vi "Main.vi"() -> ()   [LabVIEW 2021, in "Sound Manager.lvlib"]
uses:
  Sound Manager.lvlib
  Typedefs/Sound Effects.ctl
  Typedefs/States.ctl
  Typedefs/Config.ctl
  <vilib>/sound2/lvsound2.llb/Sound Output Task ID.ctl
  <vilib>/event_ctls.llb/usereventprio.ctl
  Application/App Configuration.ctl
  Application/Application.lvclass
  Configuration/Configuration.lvlib
  SubVIs/Read Sound ConfigurationI.vi
panel:
  in  "Multicolumn Listbox":i32(listbox)
  out "Background Track":string
  in  "Stop Sound Effect":bool
  in  "Play Sound Effect":bool
  in  "Sound Effect":T1
  in  "Background music":bool
  in  "Load Config":bool
  in  "Module_Refs":T2={"ModuleName"=enum."Controller", "Queue"=refnum, "user event"=refnum, "VI Refnum"=refnum, "ShowFP"=FALSE, "StatesTracking Enabled"=FALSE}
  out "error out":errorcluster
  in  "error in (no error)":errorcluster
  out "Message":string
  in  "Stop App":bool
  in  "Stop Module":bool
  # "#Architecture\n\nPlace inside this box all visible data."
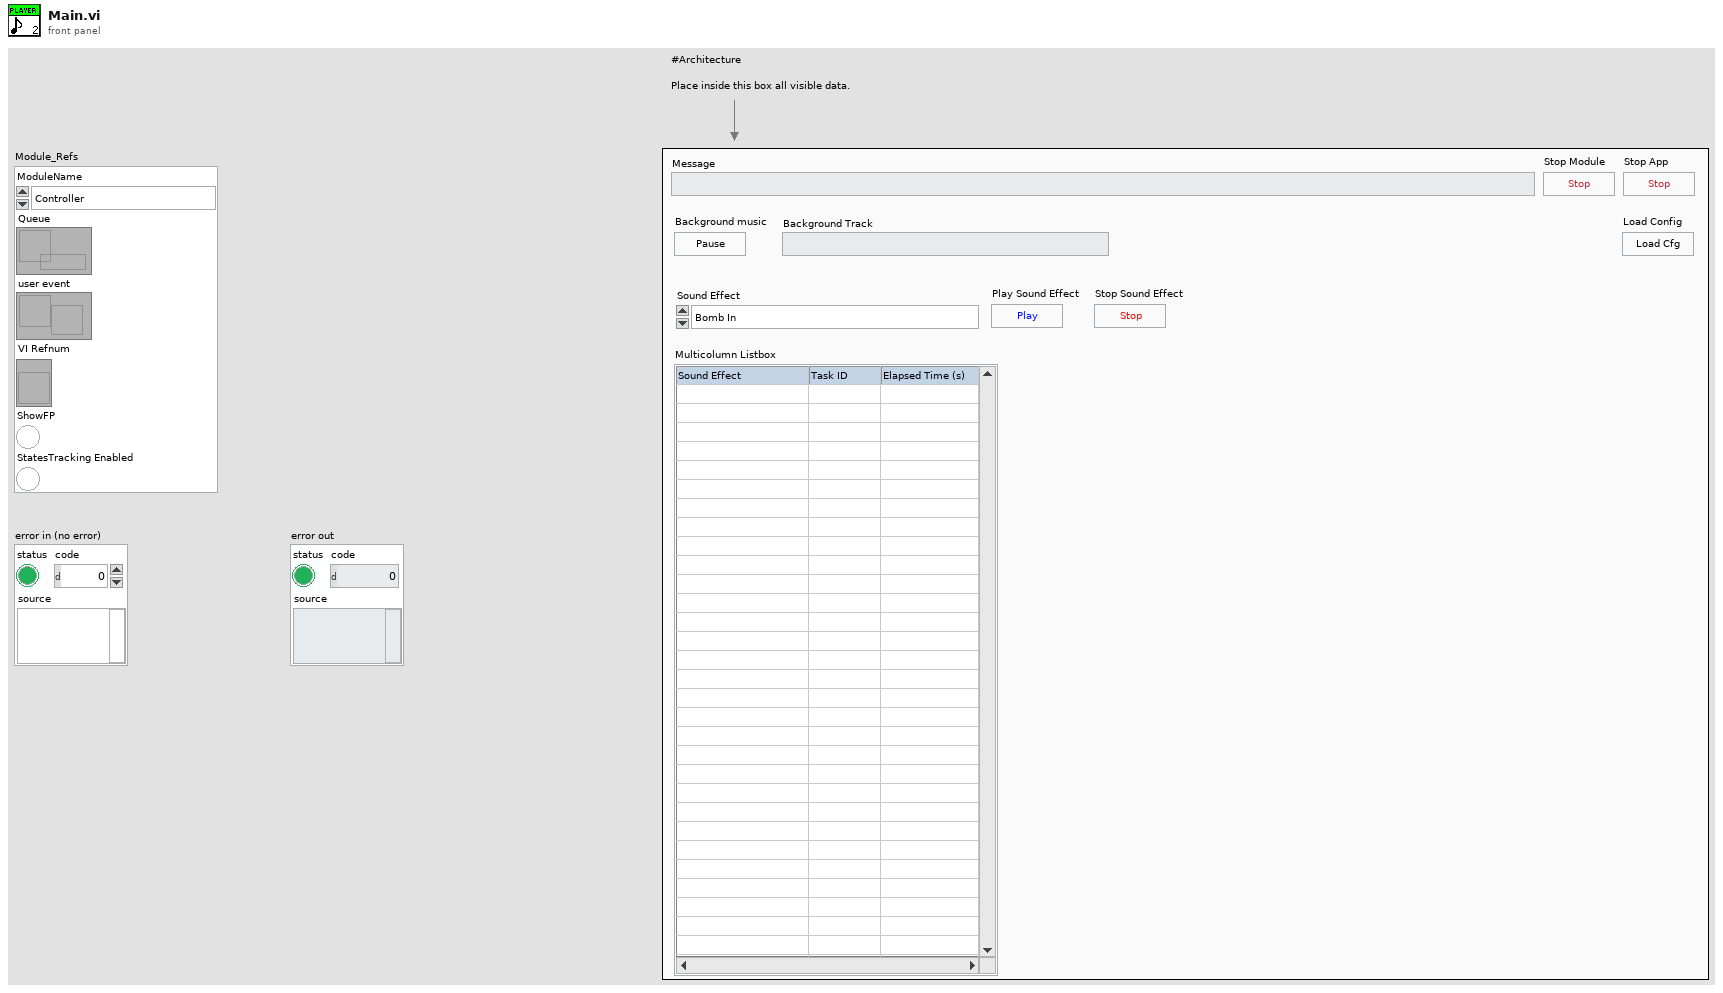
[diagram p1: front panel]
types:
  T1 = typedef "Sound Manager.lvlib/Sound Effects.ctl" = enum16{"Bomb In", "Bomb Out", "Bomb Touched", "Game Over", "Victory", "Eat", "10 Fruits", "Eat2", "Eat3", "Eat4", "MaxShield", "Shield", "10p", "Grape In", "Grape Out", "20p", "30p", "40p", "50p", "60p", "70p", "80p", "90p", "100p", "All shields cracked", "Mouse In", "Mouse Out", "Mouse Eaten", "Grape Eaten", "States Recover", "Broken Shield", "Bonus", "Happy Time", "explode", "Game over musica", "Back Music", "Shield Catch", "Evil lough", "Cricket In", "Cricket eaten", "Lets Go", "Jump1", "Jump2", "Jump3", "Unstoppable", "Troll Music", "winner"}
  T2 = typedef "Architecture.lvlib/Module References.ctl" = cluster{"ModuleName":T3, "Queue":refnum<queue>, "user event":refnum<user-event>, "VI Refnum":refnum<vi>, "ShowFP":bool, "StatesTracking Enabled":bool}
  T3 = typedef "Architecture.lvlib/Enum_Module_Name.ctl" = enum16{"Configuration", "Error_Handler", "Log", "Database", "Controller"}
  T4 = typedef "Sound Manager.lvlib/States.ctl" = cluster{"Module_Refs":T2, "Response Data":variant, "Config":T5, "Music Paused":bool, "Tasks":cluster{"Sound Effect":T1, "Task ID":T6, "Init":timestamp}[]}
  T5 = typedef "Sound Manager.lvlib/Config.ctl" = cluster{"Sound Library Path":path, "dyn sounds path":path}
  T6 = typedef "Sound Output Task ID.ctl" = u32
  T7 = enum32{"Invalid", "Standard", "Closed", "Hidden", "Minimized", "Maximized"}
  T8 = typedef "Error_Manager.lvlib/LogRotate.lvclass/LogData.ctl" = cluster{"error in":errorcluster, "replacements":string[], "Time Stamp":timestamp}
  T9 = cluster{"Sound Effect":T1, "Task ID":T6, "Init":timestamp}[]
  T10 = cluster{"Sound Effect":T1, "Task ID":T6, "Init":timestamp}
  T11 = typedef "usereventprio.ctl" = enum32{"high priority", "normal priority"}
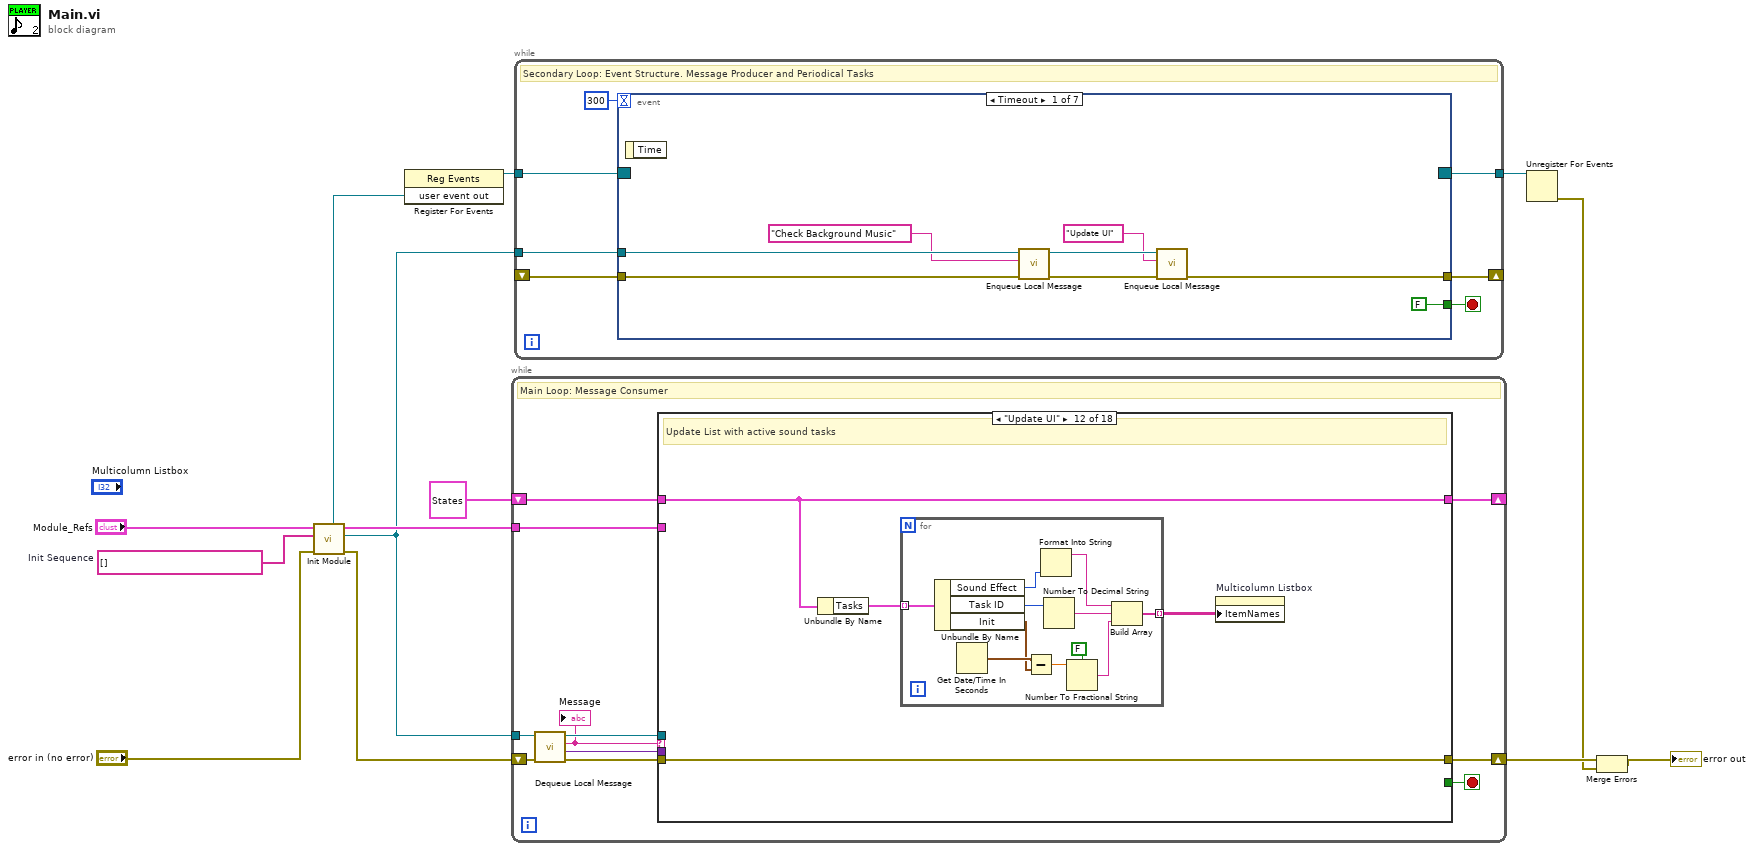
[diagram p0: block diagram]
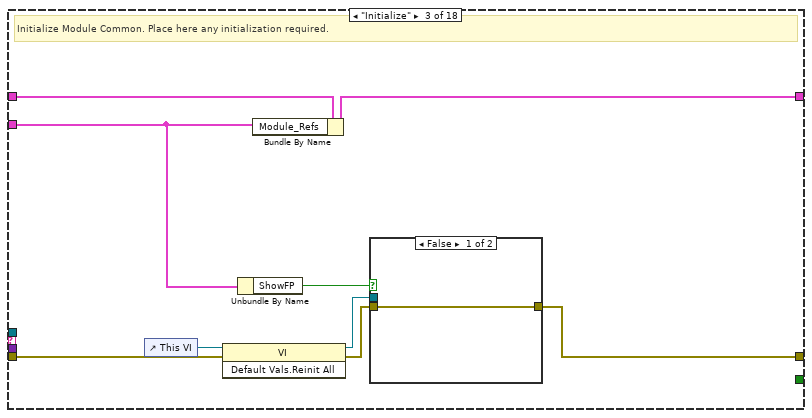
[diagram p4: hidden frame]
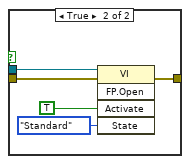
[diagram p5: hidden frame]
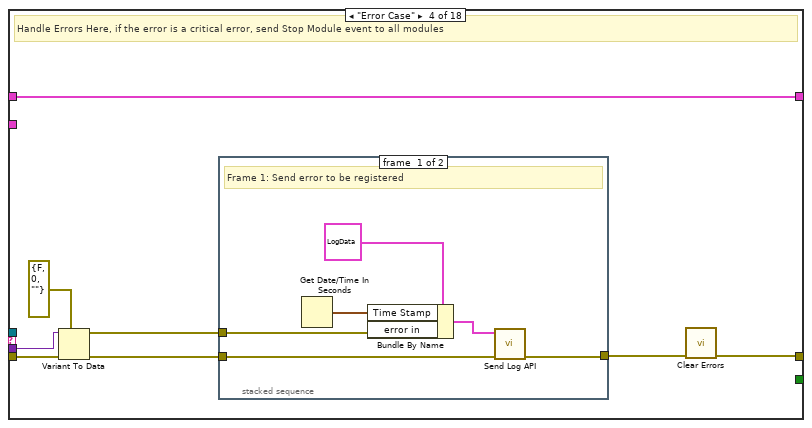
[diagram p6: hidden frame]
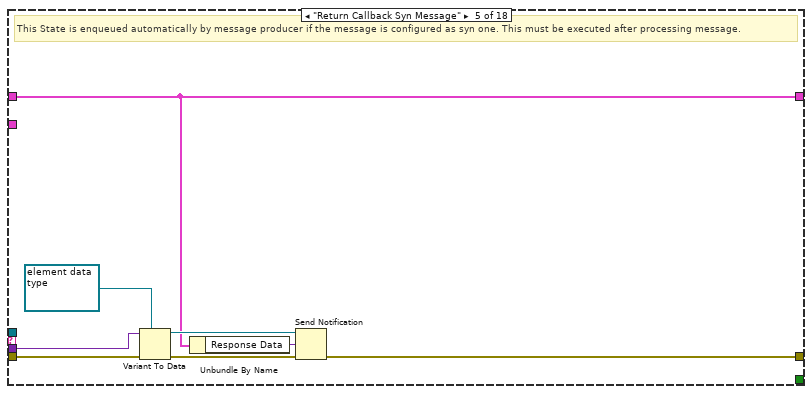
[diagram p9: hidden frame]
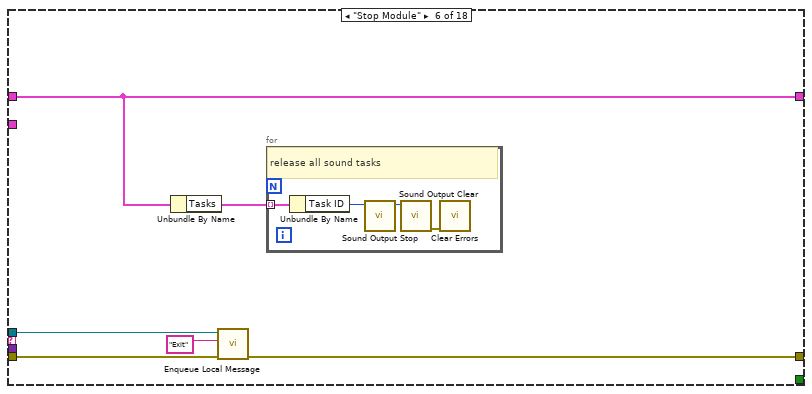
[diagram p10: hidden frame]
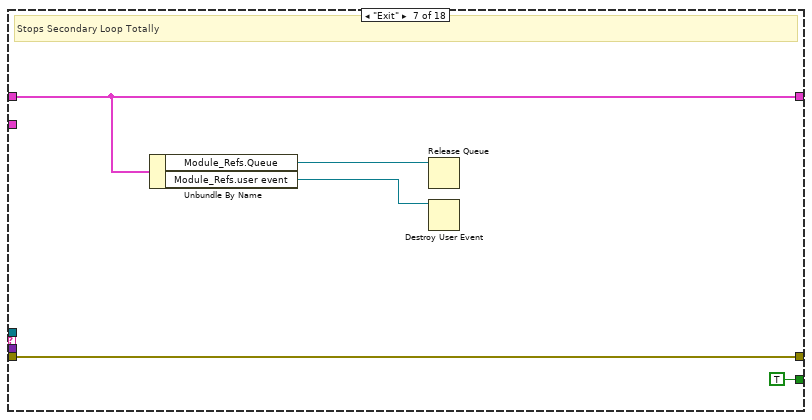
[diagram p11: hidden frame]
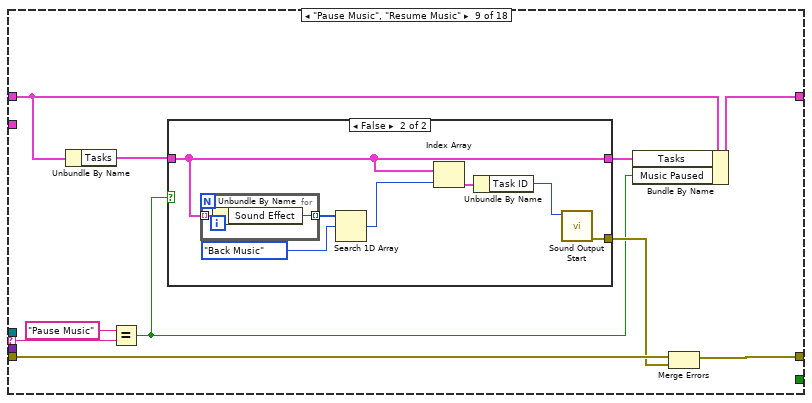
[diagram p13: hidden frame]
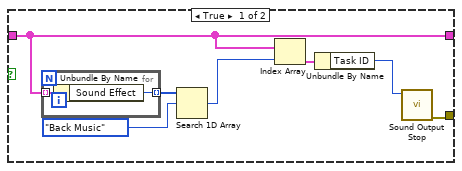
[diagram p14: hidden frame]
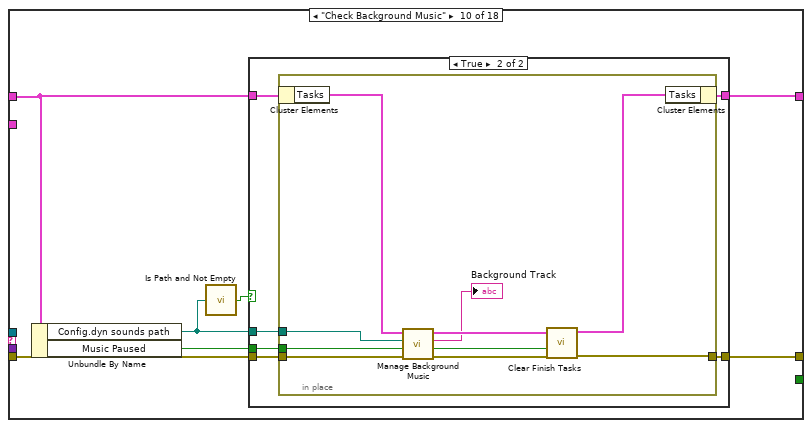
[diagram p15: hidden frame]
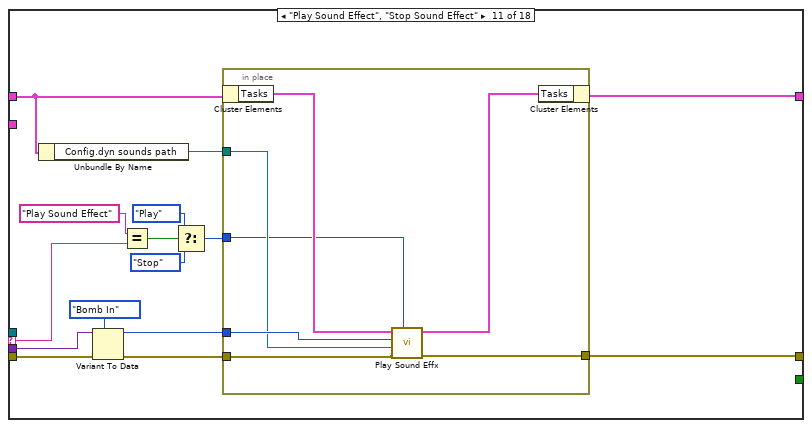
[diagram p17: hidden frame]
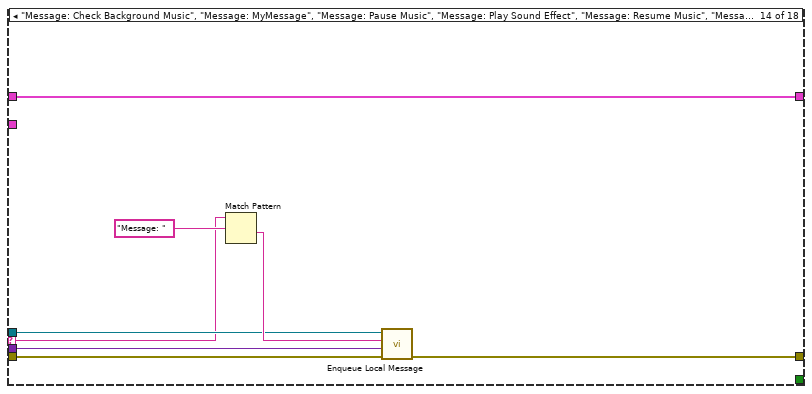
[diagram p19: hidden frame]
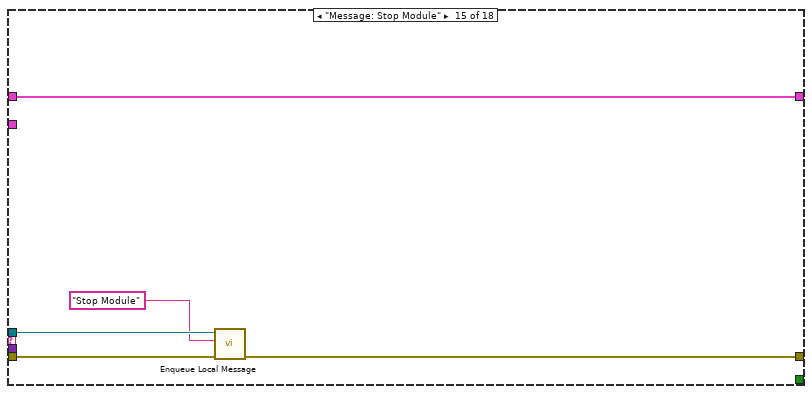
[diagram p20: hidden frame]
diagram:
  w11 = string[] []  # Init Sequence
  n1 = call "Init Module.vi"("error in (no error)"="error in (no error)", "Init Sequence"=w11, "Module Refs"="Module_Refs") -> ("error out"=w13:errorcluster, "queue out"=w2:refnum<queue>, "Module Refs Out"=w4:T2, "user event out"=w3:refnum<user-event>)  [unwired: 5 in]
  n2 = register-events(w3) -> (reference out=w10:refnum<event-registration>)  [unwired: 2 in, 1 out]
  n3 = while {
    shift-right: [w23] -> _
    shift-left: T4 {"Module_Refs"={"ModuleName"=enum."Controller", "Queue"=refnum, "user event"=refnum, "VI Refnum"=refnum, "ShowFP"=FALSE, "StatesTracking Enabled"=FALSE}, "Response Data"=variant, "Config"={"Sound Library Path"=path "", "dyn sounds path"=path ""}, "Music Paused"=FALSE, "Tasks"=[]} ("SM Data") -> [w24]
    shift-right: [w22] -> w8
    shift-left: w13 -> [w20]
    tunnel: w2 -> [w21]
    tunnel: w4 -> [w14]
    stop <- w15 stop-if-true
    # "Main Loop: Message Consumer"
    n4 = call "Dequeue Local Message.vi"("error in"=w20, "Msg queue in"=w21) -> ("error out"=w19:errorcluster, "Data"=w16:variant, "Message"=w17:string, "queue out"=w18:refnum<queue>)  [unwired: 6 in]
    "Message" <- w17
    n5 = case shown="\"Update UI\"" w17 {
      selector: w17 -> [_ _ _ _ _ _ _ _ w94 _ w144 _ _ w178 _ _ _ w222]
      tunnel: w24 -> [w26 w28 w37 w51 w63 w71 w82 w86 w92 w118 w148 w163 w177 w185 w190 w195 w213 w227]
      tunnel: [w26 w28 w35 w51 w63 w71 w82 w86 w95 w117 w146 w163 w177 w185 w190 w191 w213 w227] -> w23
      tunnel: w19 -> [w25 w27 w36 w50 w69 w75 w84 w85 w96 w120 w153 w164 w176 w182 w189 w194 w212 w226]
      tunnel: [w25 w27 w31 w44 w68 w74 w84 w85 w89 w119 w145 w164 w176 w179 w188 w192 w212 w216] -> w22
      tunnel: w18 -> [_ _ _ _ _ w73 _ _ _ _ _ _ _ w180 w187 _ _ w223]
      tunnel: w16 -> [_ _ _ w49 w66 _ _ _ _ _ w152 _ _ w181 _ w193 _ w224]
      tunnel: [_ _ _ _ _ _ TRUE _ _ _ _ _ _ _ _ _ _ _] -> w15
      tunnel: w14 -> [_ _ w34 _ _ _ _ _ _ _ _ _ _ _ _ _ _ _]
      frame "--------State Machine Arquitechture Operations--------" {
      }
      frame "Idle", Default {
        # "Use this state to make iterations if required."
      }
      frame "Initialize" {
        # "Initialize Module Common. Place here any initialization required."
        n6 = control-ref of="This VI"() -> (w29:refnum<vi>)
        n7 = invoke class="VI" method="Default Vals.Reinit All"(reference=w29, error in=w36) -> (reference out=w32:refnum<vi>, error out=w33:errorcluster)  [unwired: 1 in, 1 out]
        n8 = Unbundle By Name(w34) -> ("ShowFP"=w30:bool)
        n9 = Bundle By Name(cluster=w37, "Module_Refs"=w34) -> (w35:T4)
        n10 = case shown="False" w30 {
          tunnel: w33 -> [w38 w43]
          tunnel: [w38 w42] -> w31
          tunnel: w32 -> [_ w41]
          frame False {
          }
          frame True {
            n11 = invoke class="VI" method="FP.Open"(reference=w41, error in=w43, "Activate"=TRUE ("Activate?"), "State"=T7."Standard") -> (error out=w42:errorcluster)  [unwired: 1 in, 4 out]
          }
        }
      }
      frame "Error Case" {
        # "Handle Errors Here, if the error is a critical error, send Stop Module event to all modules"
        n12 = Variant To Data(error in=w50, type=errorcluster {"status"=FALSE, "code"=0, "source"=""} ("error constant"), Variant=w49) -> (data=w45:errorcluster, error out=w47:errorcluster)
        n13 = stacked-sequence {
          tunnel: w47 -> [w57 w59]
          tunnel: [w56 _] -> w46
          tunnel: w45 -> [w54 w58]
          frame #0 {
            # "Frame 1: Send error to be registered"
            n14 = Get Date/Time In Seconds() -> (seconds since 1Jan1904=w53:timestamp)
            n15 = Bundle By Name(cluster=T8 {"error in"={"status"=FALSE, "code"=0, "source"=""}, "replacements"=[], "Time Stamp"=timestamp(0 s since 1904-01-01)} ("Data"), "Time Stamp"=w53, "error in"=w54) -> (w52:T8)
            n16 = call "Send Log API.vi"("error in (no error)"=w57, "Data"=w52) -> ("error out"=w56:errorcluster)  [unwired: 9 in]
          }
          frame #1 {
            # "Frame 2: Manage your errors here"
            n17 = case shown="Error .." w58 {
              tunnel: [w60 w61] -> _
              tunnel: w59 -> [w60 w61]
              frame No Error {
              }
              frame Error {
                # "#Architecture \n\nPlace here critical errors to be managed \nin the desired way."
              }
            }
          }
        }
        n18 = call <vilib>:"Clear Errors.vi"("error in (no error)"=w46) -> ("error out"=w44:errorcluster)  [unwired: 5 in, 1 out]
      }
      frame "Return Callback Syn Message" {
        # "This State is enqueued automatically by message producer if the message is configured as syn one. This must be executed after processing message."
        n19 = Variant To Data(error in=w69, type=refnum<notifier> refnum ("notifier out"), Variant=w66) -> (data=w64:refnum<notifier>, error out=w67:errorcluster)
        n20 = Unbundle By Name(w63) -> ("Response Data"=w62:variant)
        n21 = Send Notification(notification=w62, notifier=w64, error in (no error)=w67) -> (error out=w68:errorcluster)  [unwired: 1 out]
      }
      frame "Stop Module" {
        n22 = Unbundle By Name(w71) -> ("Tasks"=w70:T9)
        n23 = call "Enqueue Local Message.vi"("error in"=w75, "Message"="Exit", "Msg queue in"=w73) -> ("error out"=w74:errorcluster)  [unwired: 7 in, 1 out]
        n24 = for {
          tunnel: w70 -> [w77] mode=indexing
          # "release all sound tasks"
          n25 = Unbundle By Name(w77) -> ("Task ID"=w76:T6)
          n26 = call <vilib>:"Sound Output Stop.vi"("task ID"=w76) -> ("task ID out"=w78:T6)  [unwired: 9 in, 1 out]
          n27 = call <vilib>:"Sound Output Clear.vi"("task ID"=w78) -> ("error out"=w79:errorcluster)  [unwired: 10 in]
          n28 = call <vilib>:"Clear Errors.vi"("error in (no error)"=w79) -> ()  [unwired: 5 in, 2 out]
        }
      }
      frame "Exit" {
        # "Stops Secondary Loop Totally"
        n29 = Unbundle By Name(w82) -> ("Module_Refs.Queue"=w81:refnum<queue>, "Module_Refs.user event"=w80:refnum<user-event>)
        n30 = Release Queue(queue=w81) -> ()  [unwired: 2 in, 3 out]
        n31 = Destroy User Event(user event=w80) -> ()  [unwired: 1 in, 1 out]
      }
      frame "--------------State Machine Custom States-------------" {
      }
      frame "Pause Music", "Resume Music" {
        n32 = Unbundle By Name(w92) -> ("Tasks"=w91:T9)
        n33 = Equal?(x="Pause Music", y=w94) -> (x = y?=w87:bool)
        n34 = case shown="False" w87 {
          tunnel: w91 -> [w99 w108]
          tunnel: [w99 w108] -> w90
          tunnel: [w97 w106] -> w88
          frame True {
            n35 = for {
              tunnel: w99 -> [w105] mode=indexing
              tunnel: [w104] -> w101 mode=indexing
              n36 = Unbundle By Name(w105) -> ("Sound Effect"=w104:T1)
            }
            n37 = Search 1D Array(1D array=w101, element=Sound_Effects."Back Music") -> (index of element=w100:i32)  [unwired: 1 in]
            n38 = Index Array(array=w99, index=w100) -> (element=w103:T10)
            n39 = Unbundle By Name(w103) -> ("Task ID"=w98:T6)
            n40 = call <vilib>:"Sound Output Stop.vi"("task ID"=w98) -> ("error out"=w97:errorcluster)  [unwired: 9 in, 1 out]
          }
          frame False {
            n41 = for {
              tunnel: w108 -> [w114] mode=indexing
              tunnel: [w113] -> w110 mode=indexing
              n42 = Unbundle By Name(w114) -> ("Sound Effect"=w113:T1)
            }
            n43 = Search 1D Array(1D array=w110, element=Sound_Effects."Back Music") -> (index of element=w109:i32)  [unwired: 1 in]
            n44 = Index Array(array=w108, index=w109) -> (element=w112:T10)
            n45 = Unbundle By Name(w112) -> ("Task ID"=w107:T6)
            n46 = call <vilib>:"Sound Output Start.vi"("task ID"=w107) -> ("error out"=w106:errorcluster)  [unwired: 9 in, 1 out]
          }
        }
        n47 = Bundle By Name(cluster=w92, "Tasks"=w90, "Music Paused"=w87) -> (w95:T4)
        n48 = Merge Errors(w96, w88) -> (w89:errorcluster)
      }
      frame "Check Background Music" {
        n49 = Unbundle By Name(w118) -> ("Config.dyn sounds path"=w116:path, "Music Paused"=w121:bool)
        n50 = call <vilib>:"Is Path and Not Empty.vi"("path"=w116) -> ("Is Path and Not Empty?"=w115:bool)  [unwired: 4 in]
        n51 = case shown="True" w115 {
          tunnel: w121 -> [_ w129]
          tunnel: w120 -> [w122 w128]
          tunnel: [w122 w127] -> w119
          tunnel: w118 -> [w123 w126]
          tunnel: [w123 w125] -> w117
          tunnel: w116 -> [_ w124]
          frame False {
          }
          frame True {
            n52 = in-place {
              in-place-border: w129 -> [w131]
              in-place-border: w128 -> [w138]
              in-place-border: [w132] -> w127
              in-place-border: w124 -> [w136]
              n53 = in-place-cluster #1(w126) -> ("Tasks"=w137:T9)
              n54 = call "Manage Background Music.vi"("error in (no error)"=w138, "Music Paused"=w131, "Dyn Sounds Path"=w136, "Sounds"=w137) -> ("error out"=w133:errorcluster, "Sounds Out"=w135:T9, "BackGround Track"=→"Background Track":string)  [unwired: 5 in]
              n55 = call "Clear Finish Tasks.vi"("error out"=w133, "Music Paused"=w131, "Sounds In"=w135) -> ("error out"=w132:errorcluster, "Sounds Out"=w134:T9)  [unwired: 7 in]
              n56 = in-place-cluster #1("Tasks"=w134) -> (w125:T4)
            }
          }
        }
      }
      frame "Play Sound Effect", "Stop Sound Effect" {
        n57 = Unbundle By Name(w148) -> ("Config.dyn sounds path"=w147:path)
        n58 = Variant To Data(error in=w153, type=Sound_Effects."Bomb In" ("Sound Effect"), Variant=w152) -> (data=w149:T1, error out=w150:errorcluster)
        n59 = Equal?(x="Play Sound Effect", y=w144) -> (x = y?=w142:bool)
        n60 = Select(t=enum16{"Play", "Stop"}."Play" ("event"), s=w142, f=enum16{"Play", "Stop"}."Stop" ("event")) -> (s? t:f=w139:enum16{"Play", "Stop"})
        n61 = in-place {
          in-place-border: w150 -> [w160]
          in-place-border: w149 -> [w157]
          in-place-border: w147 -> [w156]
          in-place-border: [w155] -> w145
          in-place-border: w139 -> [w154]
          n62 = in-place-cluster #2(w148) -> ("Tasks"=w158:T9)
          n63 = call "Play Sound Effx.vi"("event"=w154, "error in (no error)"=w160, "path"=w156, "Sound Effect Off"=w157, "Sounds In"=w158) -> ("error out"=w155:errorcluster, "Sounds Out"=w159:T9)  [unwired: 5 in]
          n64 = in-place-cluster #2("Tasks"=w159) -> (w146:T4)
        }
      }
      frame "Update UI" {
        # "Update List with active sound tasks"
        n65 = Unbundle By Name(w163) -> ("Tasks"=w162:T9)
        n66 = for {
          tunnel: w162 -> [w175] mode=indexing
          tunnel: [w165] -> w161 mode=indexing
          n67 = Unbundle By Name(w175) -> ("Sound Effect"=w174:T1, "Task ID"=w172:T6, "Init"=w169:timestamp)
          n68 = Get Date/Time In Seconds() -> (seconds since 1Jan1904=w170:timestamp)
          n69 = Subtract(x=w170, y=w169) -> (x-y=w168:dbl)
          n70 = Format Into String(w174) -> (resulting string=w173:string)  [unwired: 3 in, 1 out]
          n71 = Number To Decimal String(number=w172) -> (decimal integer string=w171:string)  [unwired: 1 in]
          n72 = Number To Fractional String(use system decimal point (T)=FALSE, number=w168) -> (F-format string=w166:string)  [unwired: 2 in]
          n73 = Build Array(w173, w171, w166) -> (w165:string[])
        }
        n74 = property on="Multicolumn Listbox" class="MCListbox (strict)"("ItemNames"=w161) -> ()  [unwired: 2 in, 2 out]
      }
      frame "--------------Dynamic Events Messages----------------" {
      }
      frame "Message: Check Background Music", "Message: MyMessage", "Message: Pause Music", "Message: Play Sound Effect", "Message: Resume Music", "Message: Stop Sound Effect" {
        n75 = Match Pattern(string=w178, regular expression="Message: ") -> (after substring=w183:string)  [unwired: 1 in, 3 out]
        n76 = call "Enqueue Local Message.vi"("error in"=w182, "Data"=w181, "Message"=w183, "Msg queue in"=w180) -> ("error out"=w179:errorcluster)  [unwired: 6 in, 1 out]
      }
      frame "Message: Stop Module" {
        n77 = call "Enqueue Local Message.vi"("error in"=w189, "Message"="Stop Module", "Msg queue in"=w187) -> ("error out"=w188:errorcluster)  [unwired: 7 in, 1 out]
      }
      frame "Message: Load Config" {
        # "Message used to receive configuration from a configuration module. Decode dedicated typedef and save it into SM Data"
        n78 = disable-structure shown="Simulation==True" {
          disable-tunnel: w195 -> [w204 w210]
          disable-tunnel: w194 -> [w203 w211]
          disable-tunnel: w193 -> [w202 _]
          disable-tunnel: [w196 _] -> w192
          disable-tunnel: [_ w211] -> _
          disable-tunnel: [w201 w209] -> w191
          frame condition #0 {
            n79 = Variant To Data(error in=w203, type=refnum<data-value> refnum ("data value reference"), Variant=w202) -> (data=w199:refnum<data-value>, error out=w197:errorcluster)
            n80 = call-poly "Poly Read Config API.vi"("error constant"=w197, "data value reference"=w199) -> ("error out"=w196:errorcluster, "Sound Manager Config"=w198:T5)  [unwired: 8 in]
            n81 = Bundle By Name(cluster=w204, "Config"=w198) -> (w201:T4)
          }
          frame condition #1 (active) {
            n82 = call <vilib>:"Application Directory.vi"() -> ("Application Directory"=w208:path)
            n83 = Build Path(base path=w208, name or relative path=path "Resources/sounds/%s.wav") -> (appended path=w206:path)
            n84 = Strip Path(path=w206) -> (stripped path=w205:path)  [unwired: 1 out]
            n85 = Bundle By Name(cluster=w210, "Config.Sound Library Path"=w205, "Config.dyn sounds path"=w206) -> (w209:T4)
          }
        }
      }
      frame "------------Synchronous Event Messages--------------" {
      }
      frame "SynMessage: MySynMessage" {
        # "Use this case as a handler for Synchronous messages. This state queues a message for the desired"
        n86 = call "Extract Synchronous Data.vi"("error in 2"=w226, "Variant"=w224) -> ("error in"=w225:errorcluster, "Data Out"=w219:variant, "notifier out"=w214:refnum<notifier>)  [unwired: 7 in]
        n87 = Match Pattern(string=w222, regular expression="SynMessage: ") -> (after substring=w220:string)  [unwired: 1 in, 3 out]
        n88 = call "Enqueue Local Message.vi"("error in"=w225, "Data"=w219, "Message"=w220, "Msg queue in"=w223) -> ("error out"=w218:errorcluster, "queue out"=w217:refnum<queue>)  [unwired: 6 in]
        n89 = call "Enqueue Local Message.vi"("error in"=w218, "Data"=w214, "Message"="Return Callback Syn Message", "Msg queue in"=w217) -> ("error out"=w216:errorcluster)  [unwired: 6 in, 1 out]
      }
    }
  }
  n90 = while {
    tunnel: w10 -> [w234]
    tunnel: w2 -> [w231]
    tunnel: [w230] -> w9
    shift-right: [w228] -> _
    shift-left: _ -> [w229]
    stop <- w232 stop-if-true
    # "Secondary Loop: Event Structure. Message Producer and Periodical Tasks"
    n91 = event shown="[0] Timeout" {
      selector: w234 -> [_ _ _ _ _ _ _]
      dyn-events: [_ _ _ _ _ _ _] -> w230
      timeout: 300 -> [_ _ _ _ _ _ _]
      tunnel: [FALSE w249 TRUE _ _ _ _] -> w232
      tunnel: w231 -> [w240 w254 w256 _ _ _ _]
      tunnel: w229 -> [w241 w253 w259 w261 w270 w278 w286]
      tunnel: [w235 w252 w257 w260 w269 w277 w285] -> w228
      event Timeout {
        n92 = event-data() -> ()  [unwired: 1 in, 1 out]
        n93 = call "Enqueue Local Message.vi"("error in"=w241, "Message"="Check Background Music", "Msg queue in"=w240) -> ("error out"=w238:errorcluster, "queue out"=w237:refnum<queue>)  [unwired: 7 in]
        n94 = call "Enqueue Local Message.vi"("error in"=w238, "Message"="Update UI", "Msg queue in"=w237) -> ("error out"=w235:errorcluster)  [unwired: 7 in, 1 out]
      }
      event User Event {
        # "Send message to local queue. \n(Message Consumer)"
        # "Processes an external event and enqueues a message to the local queue. It can be synchronous (with response) or NOT."
        n95 = event-data() -> ("syn"=w246:bool, "Message"=w248:string, "Data"=w251:variant)  [unwired: 1 in]
        n96 = Select(t="SynMessage: " ("string"), s=w246, f="Message: " ("string")) -> (s? t:f=w243:string)
        n97 = Concatenate Strings(w243, w248) -> (w250:string)
        n98 = call "Enqueue Local Message.vi"("error in"=w253, "Data"=w251, "Message"=w250, "Msg queue in"=w254) -> ("error out"=w252:errorcluster)  [unwired: 6 in, 1 out]
        n99 = Equal?(x=w248, y="Stop Module") -> (x = y?=w249:bool)
      }
      event "Stop Module": Value Change {
        n100 = event-data() -> ()  [unwired: 1 in, 1 out]
        n101 = call "Enqueue Local Message.vi"("error in"=w259, "Message"="Stop Module", "Msg queue in"=w256) -> ("error out"=w257:errorcluster)  [unwired: 7 in, 1 out]
      }
      event "Stop App": Value Change {
        w263 = TRUE  # All Modules
        # "Send Stop To All Modules"
        n102 = event-data() -> ()  [unwired: 1 in, 1 out]
        n103 = call "Send Message Modules.vi"("All Modules"=w263, "Error In"=w261, "Message"="Stop Module") -> ("error in (no error)"=w260:errorcluster)  [unwired: 8 in]
      }
      event "Load Config": Value Change {
        n104 = event-data() -> ()  [unwired: 1 in, 1 out]
        n105 = To Variant(anything=refnum<data-value> refnum ("data value reference")) -> (Variant=w266:variant)
        n106 = call "Send Message Module.vi"("priority (normal)"=usereventprio."high priority", "Error In"=w270, "Data"=w266, "Message"="Load Config", "Target ModuleName In"=Enum_Module_Name."Controller") -> ("error in (no error)"=w269:errorcluster)  [unwired: 6 in]
      }
      event "Background music": Value Change {
        n107 = event-data() -> ("NewVal"=w274:bool)  [unwired: 1 in]
        n108 = Select(t="Pause Music", s=w274, f="Resume Music") -> (s? t:f=w271:string)
        n109 = call "Send Message Module.vi"("priority (normal)"=usereventprio."normal priority", "Error In"=w278, "Message"=w271, "Target ModuleName In"=Enum_Module_Name."Controller") -> ("error in (no error)"=w277:errorcluster)  [unwired: 7 in]
      }
      event "Play Sound Effect", "Stop Sound Effect": Value Change {
        n110 = event-data() -> ("CtlRef"=w282:refnum<vi>)  [unwired: 1 in]
        n111 = property class="Bool"(reference=w282) -> ("Label.Text"=w281:string)  [unwired: 1 in, 2 out]
        n112 = To Variant(anything="Sound Effect") -> (Variant=w279:variant)
        n113 = call "Send Message Module.vi"("priority (normal)"=usereventprio."normal priority", "Error In"=w286, "Data"=w279, "Message"=w281, "Target ModuleName In"=Enum_Module_Name."Controller") -> ("error in (no error)"=w285:errorcluster)  [unwired: 6 in]
      }
    }
  }
  n114 = Unregister For Events(event registration refnum=w9) -> (error out=w7:errorcluster)  [unwired: 1 in]
  n115 = Merge Errors(w8, w7) -> (→"error out":errorcluster)
